vi "check-sleep.vi"(1 "wake-up timestamp":timestamp) -> (0 "dt":u32)   [LabVIEW 2021]
panel:
  out "current time":timestamp
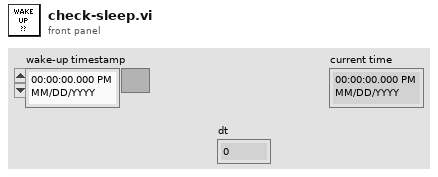
[diagram p1: front panel]
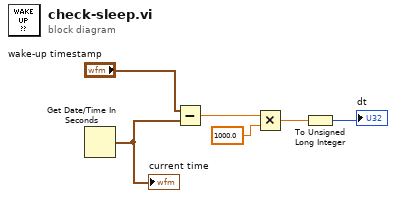
[diagram p0: block diagram]
diagram:
  n1 = Get Date/Time In Seconds() -> (seconds since 1Jan1904=w2:timestamp)
  "current time" <- w2
  n2 = Subtract(x="wake-up timestamp", y=w2) -> (x-y=w6:dbl)
  n3 = Multiply(x=w6, y=1000.0) -> (x*y=w4:dbl)
  n4 = To Unsigned Long Integer(number=w4) -> (unsigned 32bit integer=→"dt":u32)
